vi "Test JUnit with loop.vi"(8 "error in (no error)":errorcluster) -> (0 "error out":errorcluster)   [LabVIEW 2013]
uses:
  <vilib>/xml/Load XML File.vi
  classes/Assert/Assert Not Error.vi
  classes/Assert/Assert Equal Value_Variant.vi
  classes/Test Runner.Folder/Test Runner.Folder.lvclass
  classes/Test Report.JUnit/Test Report.JUnit.lvclass
  classes/Test Runner/Test Runner.lvclass
  <vilib>/xml/NI_XML.lvlib
  classes/Assert/Assert.lvclass
  classes/Test/Test.lvclass
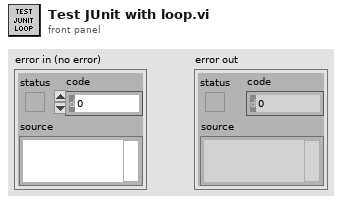
[diagram p1: front panel]
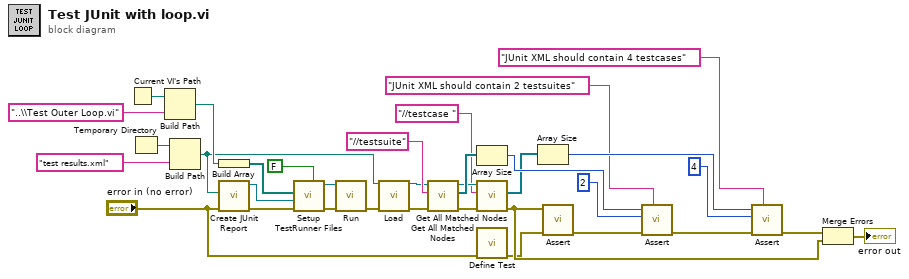
[diagram p0: block diagram]
diagram:
  n1 = Current VI's Path() -> (path=w34:path)
  n2 = Temporary Directory() -> (w28:path)
  n3 = Build Path(base path=w34, name or relative path="..\\Test Outer Loop.vi") -> (appended path=w32:path)
  n4 = Build Path(base path=w28, name or relative path="test results.xml") -> (appended path=w24:path)
  n5 = Build Array(w32) -> (w31:path[])
  n6 = call "Create JUnit Report.vi"("error in (no error)"="error in (no error)", "Report Path"=w24) -> ("error out"=w10:errorcluster, "Test Report.JUnit out"=w30:refnum<class "Test Report.JUnit.lvclass">)  [unwired: 8 in]
  n7 = call "Setup TestRunner Files.vi"("Interactive (T)"=FALSE, "error in (no error)"=w10, "Test Report"=w30, "Paths"=w31) -> ("error out"=w9:errorcluster, "Test Runner.Folder out"=w27:refnum<class "Test Runner.Folder.lvclass">)  [unwired: 6 in]
  n8 = call "Run.vi"("error in (no error)"=w9, "Test Runner in"=w27) -> ("error out"=w26:errorcluster)  [unwired: 8 in, 1 out]
  n9 = call-poly <vilib>:"Load.vi"("path to XML document"=w24, "error in (no error)"=w26) -> ("DOM document out"=w23:refnum<k20>, "error out"=w8:errorcluster)  [unwired: 11 in, 1 out]
  n10 = call <vilib>:"Get All Matched Nodes.vi"("error in (no error)"=w8, "XPath expression"="//testsuite", "node in"=w23) -> ("error out"=w18:errorcluster, "node result array"=w22:refnum<k20>[], "node out"=w19:refnum<k20>)  [unwired: 6 in]
  n11 = Array Size(array=w22) -> (size(s)=w21:i32)
  n12 = call <vilib>:"Get All Matched Nodes.vi"("error in (no error)"=w18, "XPath expression"="//testcase ", "node in"=w19) -> ("error out"=w5:errorcluster, "node result array"=w14:refnum<k20>[])  [unwired: 6 in, 1 out]
  n13 = call "Define Test.vi"("error in (no error)"="error in (no error)") -> ("error out"=w4:errorcluster)  [unwired: 10 in]
  n14 = Array Size(array=w14) -> (size(s)=w15:i32)
  n15 = call-poly "Assert.vi"("error in (no error)"=w4, "Not Error?"=w5) -> ("error out"=w3:errorcluster)  [unwired: 9 in]
  n16 = call-poly "Assert.vi"("Label"="JUnit XML should contain 2 testsuites", "error in (no error)"=w3, "Y"=2 ("size(s)"), "X"=w21) -> ("error out"=w13:errorcluster)  [unwired: 7 in]
  n17 = call-poly "Assert.vi"("Label"="JUnit XML should contain 4 testcases", "error in (no error)"=w13, "Y"=4 ("size(s)"), "X"=w15) -> ("error out"=w11:errorcluster)  [unwired: 7 in]
  n18 = Merge Errors(w11, w5) -> (→"error out":errorcluster)
